vi "GB DoF to Draw Box.vi"(6 "Force Size to Min":bool, 8 "Integer Tolerance":dbl=0.01, 9 "Mutual Viewing Angle":dbl[](array[numeric])=[1.0, -1.6612903871170226, 0.0], 10 "Grain Growth and Geometry":T4={"Min Grain 1 Length (A)"=6.0, "Min Grain 2 Length (A)"=6.0, "Min Grain Height (A)"=90.0, "Min Grain Width (A)"=90.0, "Grain 1 Start"=-0.001, "Overlap Region (A)"=0.001}, 11 "Grain Boundary Definition":T3={"Grain 1 Orientation"=[1.0, 0.6019417241891012, 0.029651947654046266], "Grain 2 Orientation"=[1.0, 0.730727623275494, 0.2205637301176], "Twist Angle (Deg)"=0.0, "Translation Vector"=[0.0, 0.0, 0.0]}) -> (2 "Draw Box Grain 2":T2, 3 "Draw Box Grain 1":T2)   [LabVIEW 2010]
panel:
  out "Suggested Dimensions":T1
  in  "Lattice Parameter":dbl=6.615785553057252
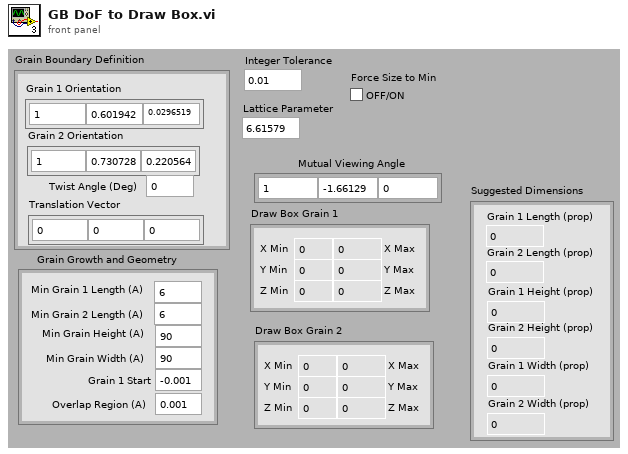
[diagram p1: front panel]
types:
  T1 = cluster{"Grain 1 Length (prop)":dbl, "Grain 2 Length (prop)":dbl, "Grain 1 Height (prop)":dbl, "Grain 2 Height (prop)":dbl, "Grain 1 Width (prop)":dbl, "Grain 2 Width (prop)":dbl}
  T2 = cluster{"X Min":dbl, "X Max":dbl, "Y Min":dbl, "Y Max":dbl, "Z Min":dbl, "Z Max":dbl}
  T3 = cluster{"Grain 1 Orientation":dbl[], "Grain 2 Orientation":dbl[], "Twist Angle (Deg)":dbl, "Translation Vector":dbl[]}
  T4 = cluster{"Min Grain 1 Length (A)":dbl, "Min Grain 2 Length (A)":dbl, "Min Grain Height (A)":dbl, "Min Grain Width (A)":dbl, "Grain 1 Start":dbl, "Overlap Region (A)":dbl}
  T5 = cluster{"Z Min":dbl, "Min Grain Width (A)":dbl, "Z Min":dbl, "Min Grain Height (A)":dbl, "Grain 1 Start":dbl, "# of Atoms":i32}
  T6 = cluster{"Z Min":dbl, "Min Grain Width (A)":dbl, "Z Min":dbl, "Min Grain Height (A)":dbl, dbl, void}
  T7 = cluster{"Grain 1 Orientation":dbl[], "Grain 2 Orientation":dbl[], "Twist Angle (Deg)":dbl}
  T8 = cluster{"Z Min":dbl, dbl, "Z Min":dbl, dbl, "Grain 1 Start":dbl, dbl}
  T9 = cluster{"Z Min":dbl, dbl, "Z Min":dbl, dbl, dbl, dbl}
  T10 = cluster{"Z Min":dbl, void, "Z Min":dbl, void, "Grain 1 Start":dbl, void}
  T11 = cluster{"Z Min":dbl, void, "Z Min":dbl, void, "Grain 1 Start":dbl, "# of Atoms":i32}
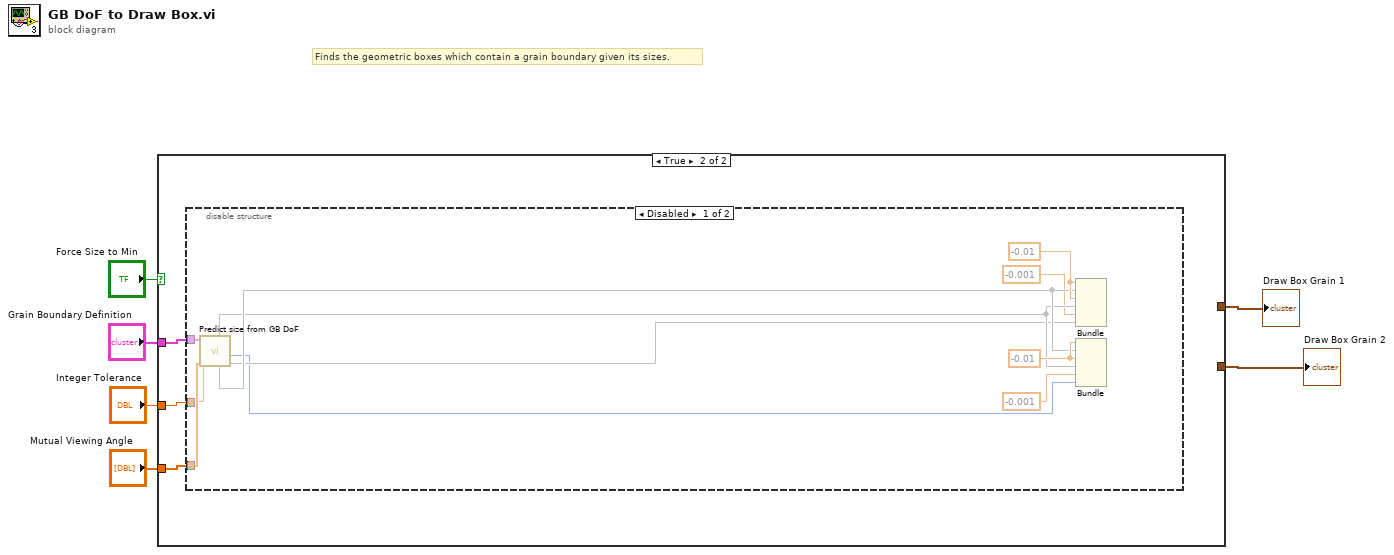
[diagram p0: block diagram]
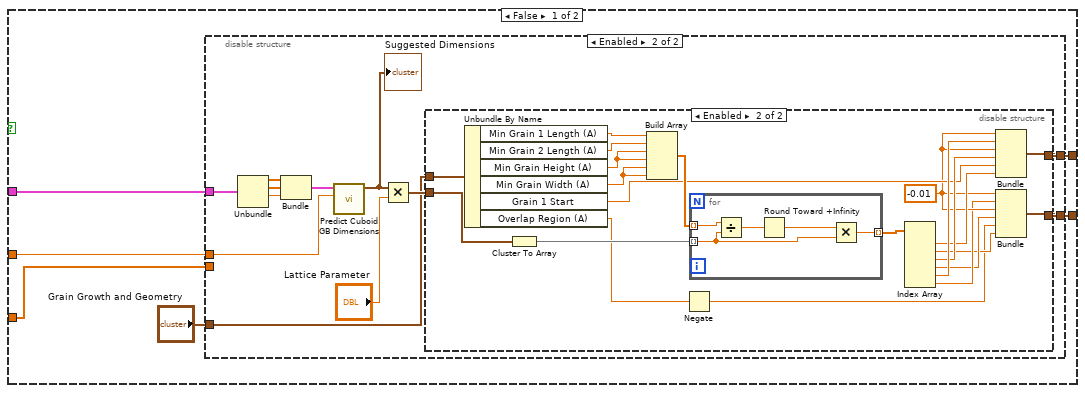
[diagram p2: hidden frame]
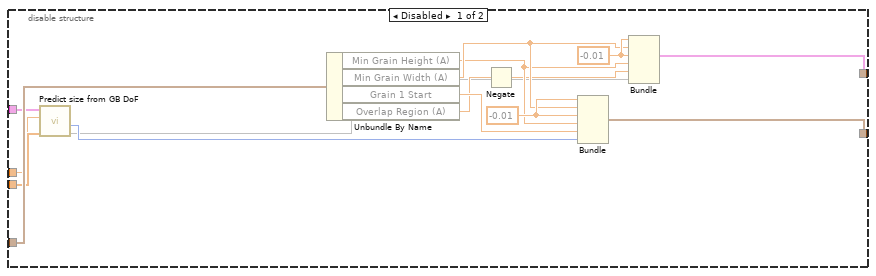
[diagram p3: hidden frame]
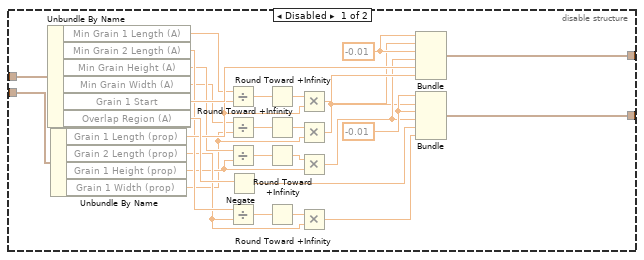
[diagram p4: hidden frame]
diagram:
  # "Finds the geometric boxes which contain a grain boundary given its sizes."
  n1 = case shown="True" "Force Size to Min" {
    tunnel: "Mutual Viewing Angle" -> [w9 w98]
    tunnel: "Grain Boundary Definition" -> [w8 w97]
    tunnel: [w11 _] -> w2
    tunnel: [w10 _] -> w3
    tunnel: "Integer Tolerance" -> [w7 w96]
    frame False {
      n2 = disable-structure shown="Enabled" {
        disable-tunnel: "Grain Growth and Geometry" -> [w28 w29]
        disable-tunnel: [w25 w30] -> w11
        disable-tunnel: [w19 w31] -> w10
        disable-tunnel: w9 -> [w18 _]
        disable-tunnel: w8 -> [w14 w39]
        disable-tunnel: w7 -> [w13 w35]
        frame Disabled {
          w24 = -0.01 ("Z Min")
          w27 = -0.01 ("Z Min")
          n3 = call "Predict size from GB DoF.vi"("Integer Tolerance"=w18, "Mutual Viewing Angle"=w13, "Grain Boundary Definition"=w14) -> (0:w16, "# of Atoms"=w17:i32, "Expected Volume (A3)"=w15:dbl)  [unwired: 5 in, 1 out]
          n4 = Unbundle By Name(w28) -> ("Min Grain Height (A)"=w22:dbl, "Min Grain Width (A)"=w23:dbl, "Grain 1 Start"=w26:dbl, "Overlap Region (A)"=w21:dbl)
          n5 = Negate(x=w21) -> (-x=w20:dbl)
          n6 = Bundle("Z Min"=w27, "Min Grain Width (A)"=w23, "Z Min"=w27, "Min Grain Height (A)"=w22, "Grain 1 Start"=w26, "# of Atoms"=w17) -> (w25:T5)  [unwired: 1 in]
          n7 = Bundle("Z Min"=w24, "Min Grain Width (A)"=w23, "Z Min"=w24, "Min Grain Height (A)"=w22, w20, w16) -> (w19:T6)  [unwired: 1 in]
        }
        frame Enabled {
          n8 = Unbundle(w39) -> ("Grain 1 Orientation"=w38:dbl[], "Grain 2 Orientation"=w37:dbl[], "Twist Angle (Deg)"=w40:dbl)  [unwired: 1 out]
          n9 = Bundle("Grain 1 Orientation"=w38, "Grain 2 Orientation"=w37, "Twist Angle (Deg)"=w40) -> (w36:T7)  [unwired: 1 in]
          n10 = call "Predict Cuboid GB Dimensions.vi"("Tolerance"=w35, "Grain Boundary Macro Definition"=w36) -> ("Suggested Cuboid Dimensions (proportional)"=w33:T1)  [unwired: 7 in, 2 out]
          "Suggested Dimensions" <- w33
          n11 = Multiply(x=w33, y="Lattice Parameter") -> (x*y=w32:T1)
          n12 = disable-structure shown="Enabled" {
            disable-tunnel: w32 -> [w69 w84]
            disable-tunnel: [w65 w77] -> w31
            disable-tunnel: [w64 w72] -> w30
            disable-tunnel: w29 -> [w41 w90]
            frame Disabled {
              w67 = -0.01 ("Z Min")
              w66 = -0.01 ("Z Min")
              n13 = Unbundle By Name(w41) -> ("Min Grain 1 Length (A)"=w61:dbl, "Min Grain 2 Length (A)"=w54:dbl, "Min Grain Height (A)"=w50:dbl, "Min Grain Width (A)"=w46:dbl, "Grain 1 Start"=w63:dbl, "Overlap Region (A)"=w62:dbl)
              n14 = Unbundle By Name(w69) -> ("Grain 1 Length (prop)"=w58:dbl, "Grain 2 Length (prop)"=w44:dbl, "Grain 1 Height (prop)"=w43:dbl, "Grain 1 Width (prop)"=w42:dbl)
              n15 = Divide(x=w61, y=w58) -> (x/y=w60:dbl)
              n16 = Divide(x=w46, y=w42) -> (x/y=w47:dbl)
              n17 = Divide(x=w50, y=w43) -> (x/y=w52:dbl)
              n18 = Divide(x=w54, y=w44) -> (x/y=w55:dbl)
              n19 = Negate(x=w62) -> (-x=w68:dbl)
              n20 = Round Toward +Infinity(x=w60) -> (ceil(x): smallest int >= x=w59:dbl)
              n21 = Round Toward +Infinity(x=w47) -> (ceil(x): smallest int >= x=w48:dbl)
              n22 = Round Toward +Infinity(x=w52) -> (ceil(x): smallest int >= x=w51:dbl)
              n23 = Round Toward +Infinity(x=w55) -> (ceil(x): smallest int >= x=w56:dbl)
              n24 = Multiply(x=w59, y=w58) -> (x*y=w57:dbl)
              n25 = Multiply(x=w48, y=w42) -> (x*y=w45:dbl)
              n26 = Multiply(x=w51, y=w43) -> (x*y=w49:dbl)
              n27 = Multiply(x=w56, y=w44) -> (x*y=w53:dbl)
              n28 = Bundle("Z Min"=w66, w45, "Z Min"=w66, w49, "Grain 1 Start"=w63, w57) -> (w65:T8)  [unwired: 1 in]
              n29 = Bundle("Z Min"=w67, w45, "Z Min"=w67, w49, w68, w53) -> (w64:T9)  [unwired: 1 in]
            }
            frame Enabled {
              w76 = -0.01 ("Z Min")
              n30 = Unbundle By Name(w90) -> ("Min Grain 1 Length (A)"=w89:dbl, "Min Grain 2 Length (A)"=w88:dbl, "Min Grain Height (A)"=w87:dbl, "Min Grain Width (A)"=w86:dbl, "Grain 1 Start"=w78:dbl, "Overlap Region (A)"=w71:dbl)
              n31 = Cluster To Array(cluster=w84) -> (array=w83:dbl[])
              n32 = Build Array(w89, w88, w87, w87, w86, w86) -> (w85:dbl[])
              n33 = Negate(x=w71) -> (-x=w70:dbl)
              n34 = for {
                tunnel: w85 -> [w93] mode=indexing
                tunnel: w83 -> [w92] mode=indexing
                tunnel: [w91] -> w82 mode=indexing
                n35 = Divide(x=w93, y=w92) -> (x/y=w95:dbl)
                n36 = Round Toward +Infinity(x=w95) -> (ceil(x): smallest int >= x=w94:dbl)
                n37 = Multiply(x=w94, y=w92) -> (x*y=w91:dbl)
              }
              n38 = Index Array(array=w82) -> (element #1=w79:dbl, element #2=w73:dbl, element #3=w80:dbl, element #4=w74:dbl, element #5=w81:dbl, element #6=w75:dbl)  [unwired: 6 in]
              n39 = Bundle("Z Min"=w76, w81, "Z Min"=w76, w80, "Grain 1 Start"=w78, w79) -> (w77:T8)  [unwired: 1 in]
              n40 = Bundle("Z Min"=w76, w75, "Z Min"=w76, w74, w70, w73) -> (w72:T9)  [unwired: 1 in]
            }
          }
        }
      }
    }
    frame True {
      n41 = disable-structure shown="Disabled" {
        disable-tunnel: w98 -> [w111 _]
        disable-tunnel: w97 -> [w110 _]
        disable-tunnel: w96 -> [w99 _]
        frame Disabled {
          w106 = -0.01 ("Z Min")
          w109 = -0.01 ("Z Min")
          n42 = call "Predict size from GB DoF.vi"("Integer Tolerance"=w111, "Mutual Viewing Angle"=w99, "Grain Boundary Definition"=w110) -> (0:w102, "# of Atoms"=w100:i32, 4:w105, 5:w104)  [unwired: 3 in, 2 out]
          n43 = Bundle("Z Min"=w106, w105, "Z Min"=w106, w104, "Grain 1 Start"=-0.001, w102) -> (w101:T10)  [unwired: 1 in]
          n44 = Bundle("Z Min"=w109, w105, "Z Min"=w109, w104, "Grain 1 Start"=-0.001, "# of Atoms"=w100) -> (w107:T11)  [unwired: 1 in]
        }
        frame Enabled {
        }
      }
    }
  }
  "Draw Box Grain 1" <- w3
  "Draw Box Grain 2" <- w2
